vi "Easy XML Editor.vi"() -> ()   [LabVIEW 2017]
doc: "A tool for editing LabVIEW objects as XML that's quicker than using the other resource editor VI."
uses:
  Resource Array.ctl
  Resource.ctl
  Find Resource by Type (String).vi
panel:
  in  "Paste FP":bool
  in  "Copy FP":bool
  in  "Front Panel XML":string
  in  "Paste BD":bool
  in  "Copy BD":bool
  in  "Block Diagram XML":string
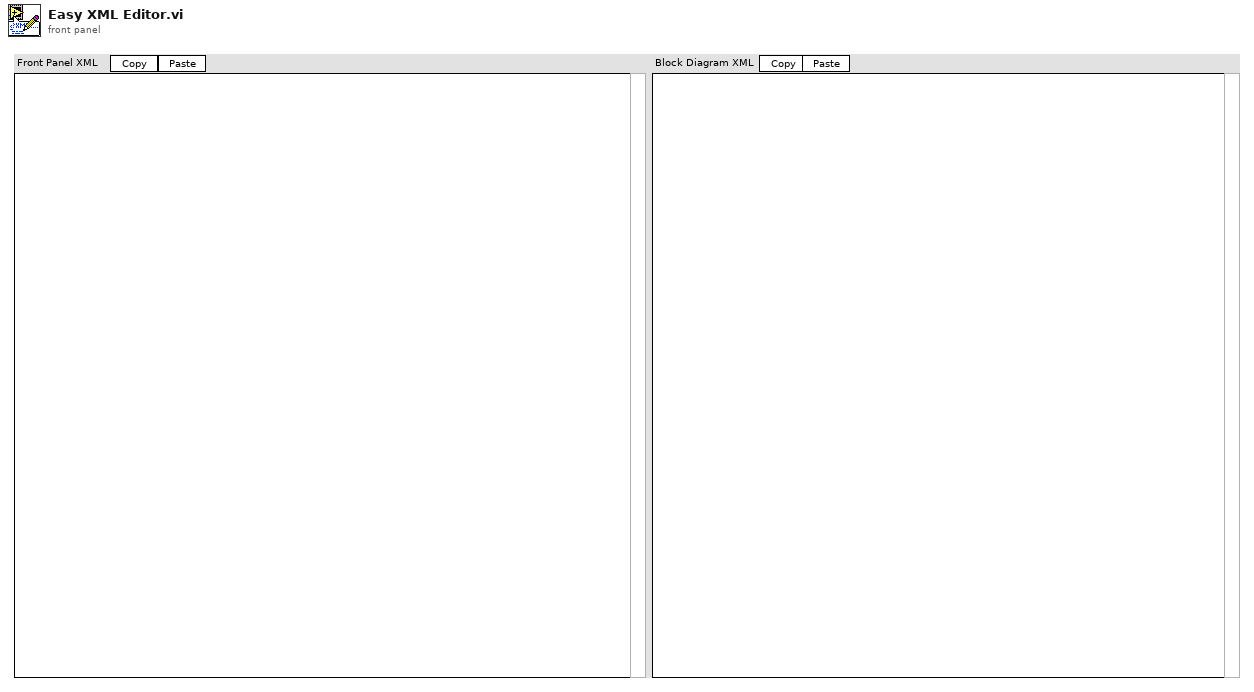
[diagram p1: front panel]
types:
  T1 = typedef "Resource Array.ctl" = T2[]
  T2 = typedef "Resource.ctl" = cluster{"type":u32, "id":i32, "name":string, "binary data":string}
  T3 = cluster{"Stored Resources":T1, "Use Stored Resources?":bool, "Last Edited VI Path":path}
  T4 = typedef "LVPositionTypeDef.ctl" = cluster{"Left":i32, "Top":i32}
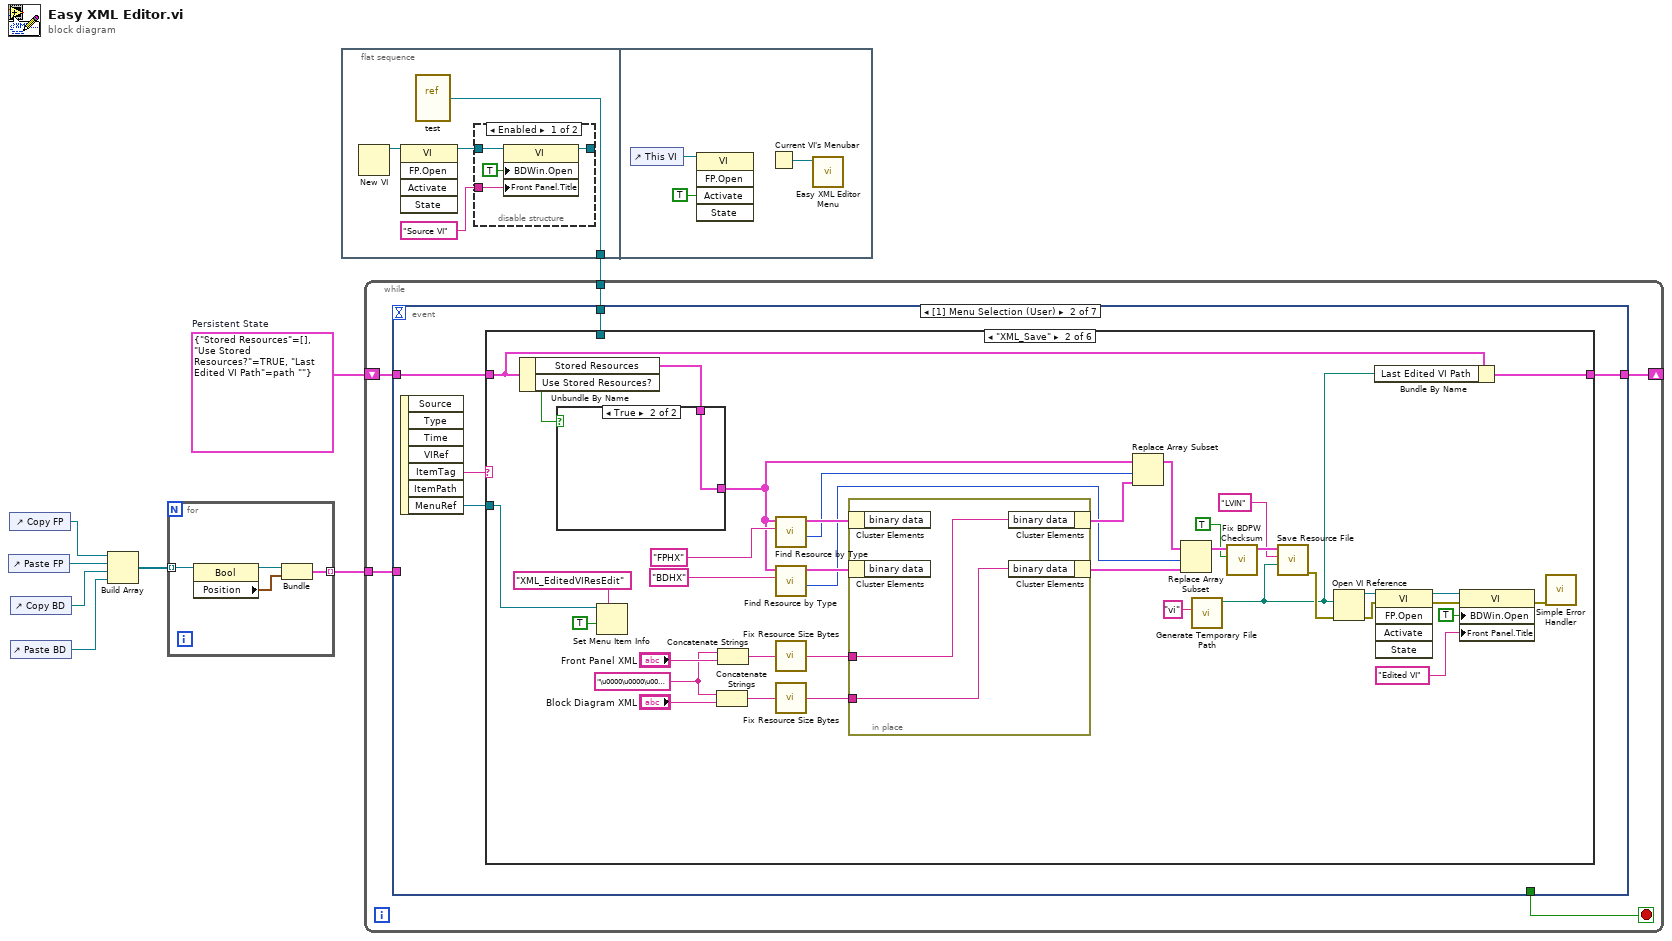
[diagram p0: block diagram]
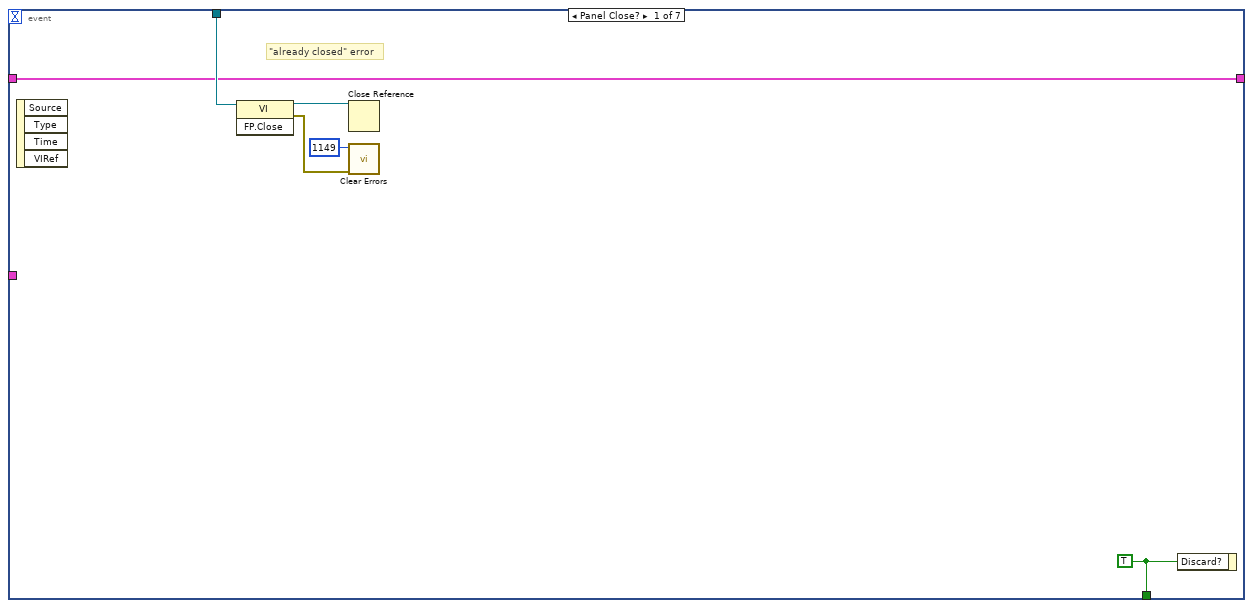
[diagram p2: hidden frame]
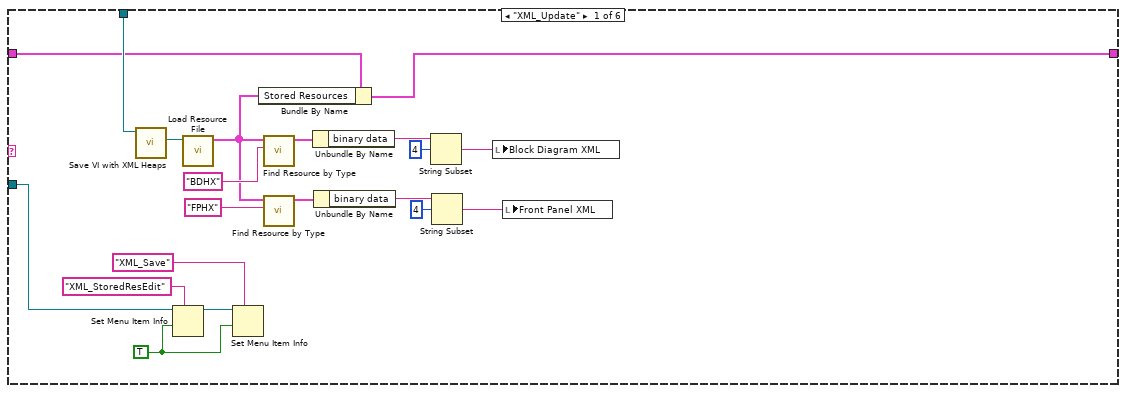
[diagram p3: hidden frame]
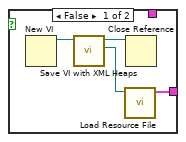
[diagram p4: hidden frame]
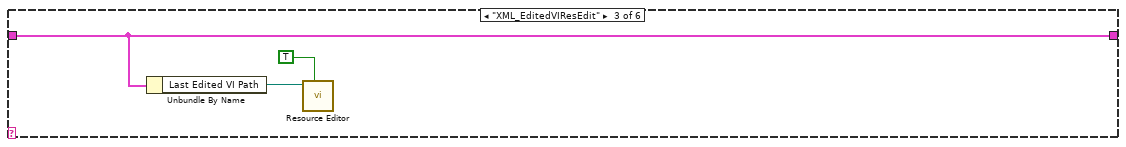
[diagram p5: hidden frame]
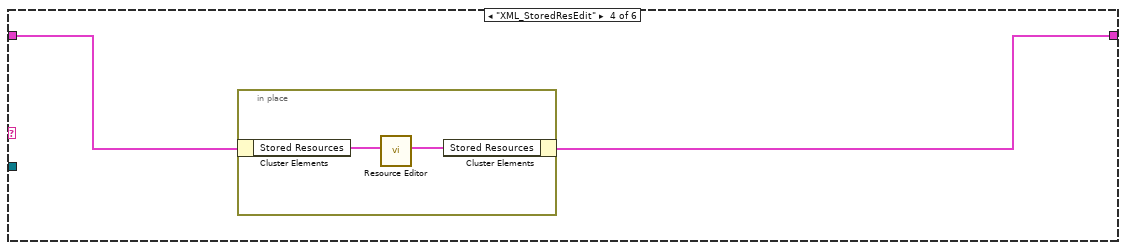
[diagram p6: hidden frame]
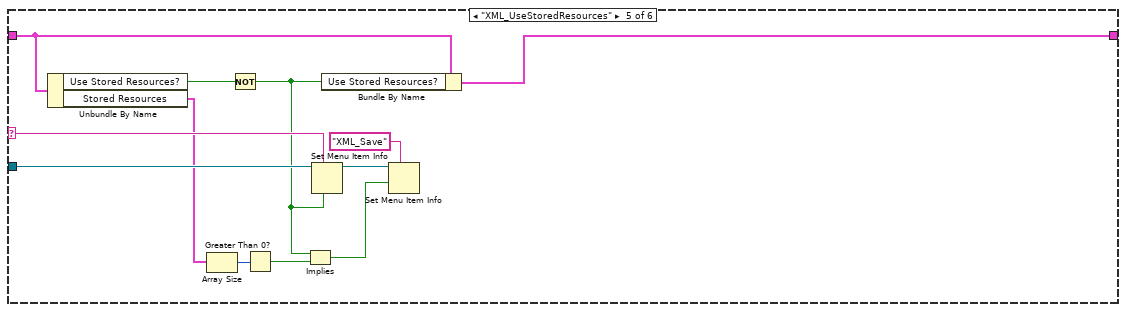
[diagram p7: hidden frame]
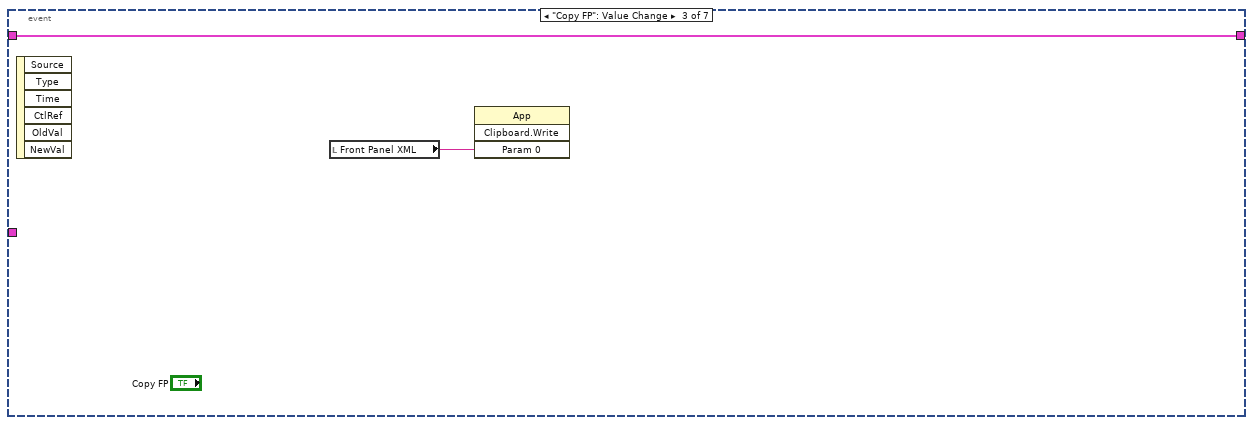
[diagram p9: hidden frame]
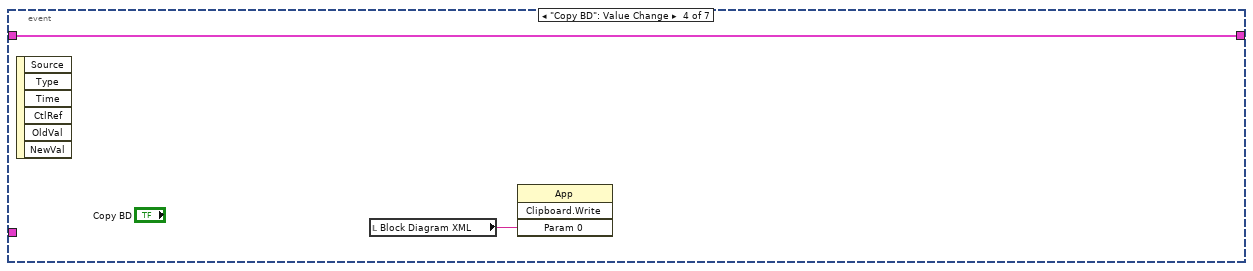
[diagram p10: hidden frame]
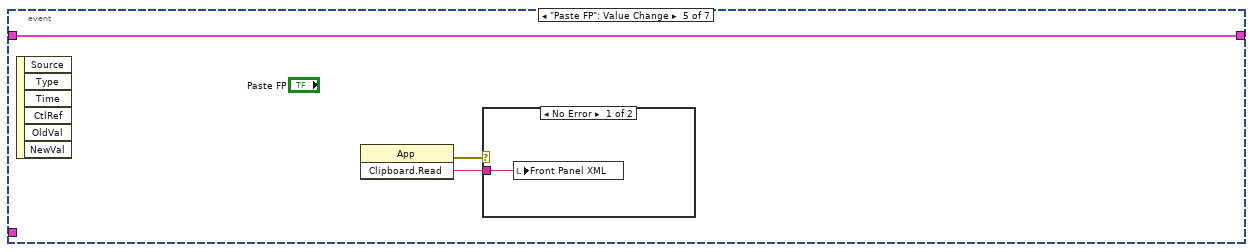
[diagram p11: hidden frame]
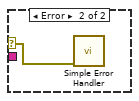
[diagram p12: hidden frame]
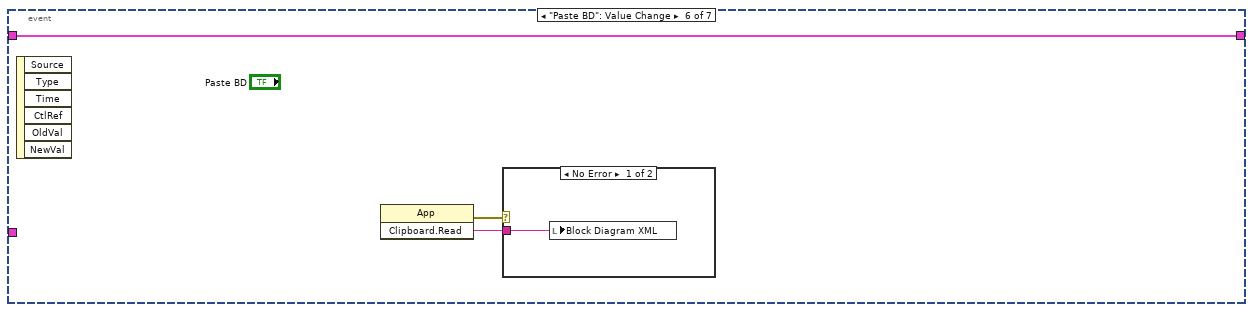
[diagram p13: hidden frame]
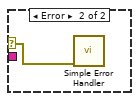
[diagram p14: hidden frame]
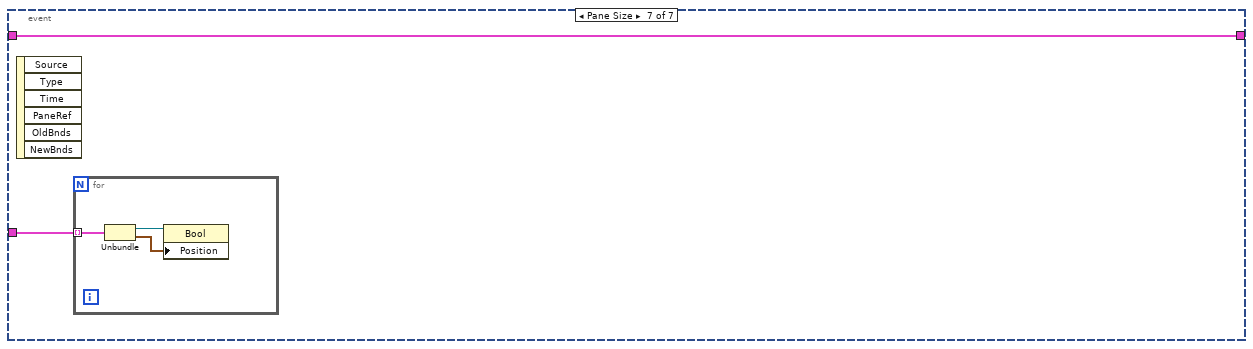
[diagram p15: hidden frame]
diagram:
  w7 = T3 {"Stored Resources"=[], "Use Stored Resources?"=TRUE, "Last Edited VI Path"=path ""}  # Persistent State
  n1 = control-ref of="Paste FP"() -> (w5:refnum<vi>)
  n2 = control-ref of="Copy FP"() -> (w6:refnum<vi>)
  n3 = control-ref of="Copy BD"() -> (w4:refnum<vi>)
  n4 = control-ref of="Paste BD"() -> (w3:refnum<vi>)
  n5 = Build Array(w6, w5, w4, w3) -> (w2:refnum<vi>[])
  n6 = for {
    tunnel: w2 -> [w12] mode=indexing
    tunnel: [w9] -> w1 mode=indexing
    n7 = property class="Bool"(reference=w12) -> (reference out=w11:refnum<vi>, "Position"=w10:T4)  [unwired: 1 in, 1 out]
    n8 = Bundle("Paste BD"=w11, "Position"=w10) -> (w9:cluster{"Paste BD":refnum<vi>, "Position":T4})  [unwired: 1 in]
  }
  n9 = flat-sequence {
    tunnel: [w13] -> w8
    frame #0 {
      n10 = New VI() -> (3:w16:refnum<vi>)  [unwired: 7 in, 1 out]
      n11 = invoke class="VI" method="FP.Open"(reference=w16) -> (reference out=w15:refnum<vi>)  [unwired: 4 in, 4 out]
      n12 = vi-ref "test.vi"() -> (w13:refnum<vi>)
      n13 = disable-structure shown="Enabled" {
        disable-tunnel: w15 -> [w20 w21]
        disable-tunnel: [w18 w21] -> _
        disable-tunnel: "Source VI" -> [w17 _]
        frame Enabled {
          n14 = property class="VI"(reference=w20, "BDWin.Open"=TRUE ("Block Diagram Window:Open"), "Front Panel.Title"=w17) -> (reference out=w18:refnum<vi>)  [unwired: 1 in, 1 out]
        }
        frame Disabled {
        }
      }
    }
    frame #1 {
      n15 = control-ref of="This VI"() -> (w24:refnum<vi>)
      n16 = invoke class="VI" method="FP.Open"(reference=w24, "Activate"=TRUE ("Activate?")) -> ()  [unwired: 3 in, 5 out]
      n17 = Current VI's Menubar() -> (w22:refnum<k9>)
      n18 = call "Easy XML Editor Menu.vi"("Menu Refnum In"=w22) -> ()  [unwired: 9 in, 2 out]
    }
  }
  n19 = while {
    tunnel: w8 -> [w29]
    shift-right: [w26] -> _
    shift-left: w7 -> [w27]
    tunnel: w1 -> [w25]
    stop <- w28 stop-if-true
    n20 = event shown="[1] Menu Selection (User)" {
      selector: _ -> [_ _ _ _ _ _ _]
      dyn-events: _ -> [_ _ _ _ _ _ _]
      timeout: _ -> [_ _ _ _ _ _ _]
      tunnel: w29 -> [w35 w39 _ _ _ _ _]
      tunnel: [w33 _ _ _ _ _ _] -> w28
      tunnel: w27 -> [w30 w38 w126 w128 w130 w135 w140]
      tunnel: [w30 w37 w126 w128 w130 w135 w140] -> w26
      tunnel: w25 -> [_ _ _ _ _ _ w141]
      event Panel Close? {
        w33 = TRUE
        # "\"already closed\" error"
        n21 = event-data() -> ()  [unwired: 1 in, 4 out]
        n22 = invoke class="VI" method="FP.Close"(reference=w35) -> (reference out=w34:refnum<vi>, error out=w32:errorcluster)  [unwired: 2 in, 1 out]
        n23 = Close Reference(reference=w34) -> ()  [unwired: 1 in, 1 out]
        n24 = call <vilib>:"Clear Errors.vi"("error in (no error)"=w32, "specific error code to clear (0: all)"=1149) -> ()  [unwired: 4 in, 2 out]
        n25 = event-data("Discard?"=w33) -> ()  [unwired: 1 in, 1 out]
      }
      event Menu Selection (User) {
        n26 = event-data() -> ("ItemTag"=w40:string, "MenuRef"=w36:refnum<k9>)  [unwired: 1 in, 5 out]
        n27 = case shown="\"XML_Save\"" w40 {
          selector: w40 -> [_ _ _ _ w120 _]
          tunnel: w39 -> [w60 _ _ _ _ _]
          tunnel: w38 -> [w47 w66 w108 w110 w123 w125]
          tunnel: [w46 w65 w108 w109 w122 w125] -> w37
          tunnel: w36 -> [w45 w63 _ _ w121 _]
          frame "XML_Update" {
            w42 = TRUE ("enabled")
            n28 = call "Save VI with XML Heaps.vi"("VI Refnum In"=w60) -> ("VI Path out"=w59:path)  [unwired: 8 in, 2 out]
            n29 = Set Menu Item Info(7:"XML_StoredResEdit", 9:w42, 11:w45) -> (3:w43:refnum<k9>)  [unwired: 4 in, 1 out]
            n30 = call "Load Resource File.vi"("Resource file"=w59) -> ("Resources"=w48:T1)  [unwired: 8 in, 2 out]
            n31 = Set Menu Item Info(7:"XML_Save", 9:w42, 11:w43) -> ()  [unwired: 4 in, 2 out]
            n32 = Bundle By Name(cluster=w47, "Stored Resources"=w48) -> (w46:T3)
            n33 = call-poly "Find Resource by Type.vi"("Resource Type"="BDHX", "Resources"=w48) -> ("Resource"=w55:T2)  [unwired: 7 in, 2 out]
            n34 = call-poly "Find Resource by Type.vi"("Resource Type"="FPHX", "Resources"=w48) -> ("Resource"=w49:T2)  [unwired: 7 in, 2 out]
            n35 = Unbundle By Name(w55) -> ("binary data"=w58:string)
            n36 = Unbundle By Name(w49) -> ("binary data"=w50:string)
            n37 = String Subset(string=w58, offset (0)=4) -> (substring=w56:string)  [unwired: 1 in]
            n38 = String Subset(string=w50, offset (0)=4) -> (substring=w52:string)  [unwired: 1 in]
            n39 = local write "Block Diagram XML"(w56) -> ()
            n40 = local write "Front Panel XML"(w52) -> ()
          }
          frame "XML_Save" {
            w94 = "\u0000\u0000\u0000\u0000"
            n41 = Unbundle By Name(w66) -> ("Stored Resources"=w67:T1, "Use Stored Resources?"=w68:bool)
            n42 = case shown="True" w68 {
              tunnel: [w99 w103] -> w84
              tunnel: w67 -> [_ w103]
              frame False {
                n43 = New VI() -> (3:w102:refnum<vi>)  [unwired: 7 in, 1 out]
                n44 = call "Save VI with XML Heaps.vi"("VI Refnum In"=w102) -> ("VI Path out"=w100:path, "VI Refnum Out"=w101:refnum<vi>)  [unwired: 8 in, 1 out]
                n45 = call "Load Resource File.vi"("Resource file"=w100) -> ("Resources"=w99:T1)  [unwired: 8 in, 2 out]
                n46 = Close Reference(reference=w101) -> ()  [unwired: 1 in, 1 out]
              }
              frame True {
              }
            }
            n47 = Set Menu Item Info(7:"XML_EditedVIResEdit", 9:TRUE ("enabled"), 11:w63) -> ()  [unwired: 4 in, 2 out]
            n48 = Concatenate Strings(w94, "Block Diagram XML") -> (w92:string)
            n49 = Concatenate Strings(w94, "Front Panel XML") -> (w93:string)
            n50 = call-poly "Find Resource by Type.vi"("Resource Type"="FPHX", "Resources"=w84) -> ("Index"=w87:i32, "Resource"=w89:T2)  [unwired: 7 in, 1 out]
            n51 = call-poly "Find Resource by Type.vi"("Resource Type"="BDHX", "Resources"=w84) -> ("Index"=w83:i32, "Resource"=w88:T2)  [unwired: 7 in, 1 out]
            n52 = call "Fix Resource Size Bytes.vi"("Data In"=w93) -> ("Data Out"=w91:string)
            n53 = call "Fix Resource Size Bytes.vi"("Data In"=w92) -> ("Data Out"=w90:string)
            n54 = in-place {
              in-place-border: w91 -> [w105]
              in-place-border: w90 -> [w104]
              n55 = in-place-cluster #1(w89) -> ()  [unwired: 1 out]
              n56 = in-place-cluster #2(w88) -> ()  [unwired: 1 out]
              n57 = in-place-cluster #1("binary data"=w105) -> (w86:T2)
              n58 = in-place-cluster #2("binary data"=w104) -> (w85:T2)
            }
            n59 = Replace Array Subset(array=w84, new element=w86, index=w87) -> (w82:T1)
            n60 = Replace Array Subset(array=w82, new element=w85, index=w83) -> (w75:T1)
            n61 = call <vilib>:"Generate Temporary File Path.vi"("Temporary File Extension (tmp)"="vi") -> ("Unique Temporary File Path"=w64:path)  [unwired: 9 in, 1 out]
            n62 = call "Fix BDPW Checksum.vi"("Only fix 3rd hash (F)"=TRUE, "Resources in"=w75) -> ("Resources out"=w74:T1)  [unwired: 9 in]
            n63 = call "Save Resource File.vi"("Path"=w64, "File type"="LVIN", "Resources"=w74) -> ("error out"=w80:errorcluster)  [unwired: 8 in]
            n64 = Open VI Reference(vi path=w64, error in (no error)=w80) -> (vi reference=w76:refnum<vi>, error out=w72:errorcluster)  [unwired: 4 in]
            n65 = Bundle By Name(cluster=w66, "Last Edited VI Path"=w64) -> (w65:T3)
            n66 = invoke class="VI" method="FP.Open"(reference=w76, error in=w72) -> (reference out=w77:refnum<vi>, error out=w71:errorcluster)  [unwired: 3 in, 3 out]
            n67 = property class="VI"(reference=w77, error in=w71, "BDWin.Open"=TRUE ("Block Diagram Window:Open"), "Front Panel.Title"="Edited VI") -> (error out=w70:errorcluster)  [unwired: 1 out]
            n68 = call <vilib>:"Simple Error Handler.vi"("error in (no error)"=w70) -> ()  [unwired: 4 in, 5 out]
          }
          frame "XML_EditedVIResEdit" {
            n69 = Unbundle By Name(w108) -> ("Last Edited VI Path"=w107:path)
            n70 = call "Resource Editor.vi"("Load from Initial Path (F)"=TRUE, "Path"=w107) -> ()  [unwired: 9 in, 1 out]
          }
          frame "XML_StoredResEdit" {
            n71 = in-place {
              n72 = in-place-cluster #3(w110) -> ("Stored Resources"=w112:T1)
              n73 = call "Resource Editor.vi"("Initial Resources"=w112) -> ("Final Resources"=w111:T1)  [unwired: 10 in]
              n74 = in-place-cluster #3("Stored Resources"=w111) -> (w109:T3)
            }
          }
          frame "XML_UseStoredResources" {
            n75 = Unbundle By Name(w123) -> ("Use Stored Resources?"=w124:bool, "Stored Resources"=w117:T1)
            n76 = Array Size(array=w117) -> (size(s)=w115:i32)
            n77 = Not(x=w124) -> (.not. x?=w116:bool)
            n78 = Greater Than 0?(x=w115) -> (x > 0?=w114:bool)
            n79 = Implies(1:w114, 2:w116) -> (0:w113:bool)
            n80 = Set Menu Item Info(6:w116, 7:w120, 11:w121) -> (3:w119:refnum<k9>)  [unwired: 4 in, 1 out]
            n81 = Bundle By Name(cluster=w123, "Use Stored Resources?"=w116) -> (w122:T3)
            n82 = Set Menu Item Info(7:"XML_Save" ("item tag"), 9:w113, 11:w119) -> ()  [unwired: 4 in, 2 out]
          }
          frame Default {
          }
        }
      }
      event "Copy FP": Value Change {
        n83 = event-data() -> ()  [unwired: 1 in, 6 out]
        n84 = local read "Front Panel XML"() -> (w127:string)
        n85 = invoke class="App" method="Clipboard.Write"("Param 0"=w127) -> ()  [unwired: 3 in, 4 out]
      }
      event "Copy BD": Value Change {
        n86 = event-data() -> ()  [unwired: 1 in, 6 out]
        n87 = local read "Block Diagram XML"() -> (w129:string)
        n88 = invoke class="App" method="Clipboard.Write"("Param 0"=w129) -> ()  [unwired: 3 in, 4 out]
      }
      event "Paste FP": Value Change {
        n89 = event-data() -> ()  [unwired: 1 in, 6 out]
        n90 = invoke class="App" method="Clipboard.Read"() -> (error out=w131:errorcluster, "Read Clipbrd"=w132:string)  [unwired: 3 in, 1 out]
        n91 = case shown="No Error" w131 {
          selector: w131 -> [_ w134]
          tunnel: w132 -> [w133 _]
          frame No Error {
            n92 = local write "Front Panel XML"(w133) -> ()
          }
          frame Error {
            n93 = call <vilib>:"Simple Error Handler.vi"("error in (no error)"=w134) -> ()  [unwired: 4 in, 5 out]
          }
        }
      }
      event "Paste BD": Value Change {
        n94 = event-data() -> ()  [unwired: 1 in, 6 out]
        n95 = invoke class="App" method="Clipboard.Read"() -> (error out=w136:errorcluster, "Read Clipbrd"=w137:string)  [unwired: 3 in, 1 out]
        n96 = case shown="No Error" w136 {
          selector: w136 -> [_ w139]
          tunnel: w137 -> [w138 _]
          frame No Error {
            n97 = local write "Block Diagram XML"(w138) -> ()
          }
          frame Error {
            n98 = call <vilib>:"Simple Error Handler.vi"("error in (no error)"=w139) -> ()  [unwired: 4 in, 5 out]
          }
        }
      }
      event Pane Size {
        n99 = event-data() -> ()  [unwired: 1 in, 6 out]
        n100 = for {
          tunnel: w141 -> [w144] mode=indexing
          n101 = Unbundle(w144) -> ("Paste BD"=w143:refnum<vi>, "Position"=w142:T4)
          n102 = property class="Bool"(reference=w143, "Position"=w142) -> ()  [unwired: 1 in, 2 out]
        }
      }
    }
  }
